vi "FPGA_HoppingStep_2ndEd(NoXYCalculation).vi"() -> ()   [LabVIEW 2014]
uses:
  <vilib>/Platform/TimedLoop/XDataNode/timing_clust.ctl
  <vilib>/Platform/TimedLoop/XDataNode/nitl_modes.ctl
  <vilib>/Platform/TimedLoop/XDataNode/wakeup.ctl
  <vilib>/rvi/Emulation/niFpgaGetClockAttributes.vi
  <vilib>/rvi/Emulation/niFpgaSctlEmulationGetInTimedLoop.vi
  <vilib>/rvi/Emulation/niFpgaEmulationReportErrorSimple.vi
  <vilib>/rvi/interface/RandomDataEmulation/niFpgaRandomDataHandleErrors.vi
  <vilib>/rvi/eio/common/nirviEmuTemplateMethod_errors.vi
  <vilib>/rvi/Emulation/niFpgaCriticalErrorInLSC.vi
  <vilib>/rvi/Emulation/niFpgaProcessEmulError.vi
  <vilib>/rvi/DataTransferAndStorage/Container/XNode/niFpgaContainer.xnode
  <vilib>/rvi/interface/RandomDataEmulation/nirviRandomDataFpgaReadWriteTemplate.vi
  <vilib>/eio/EIONode/EIONode.xnode
  <vilib>/Platform/TimedLoop/XDataNode/XDataNode.xnode
  <vilib>/Platform/TimedLoop/XDataNode/XDNodeRunTimeDep.lvlib
panel:
  out "LastObtained":i32(graph)
  in  "stop":bool
  out "Z":i32(graph)
  out "ZPresPos":i16
  in  "Sleep us":i16
  in  "RelativeWithdraw":i16
  in  "ZOffset":i16
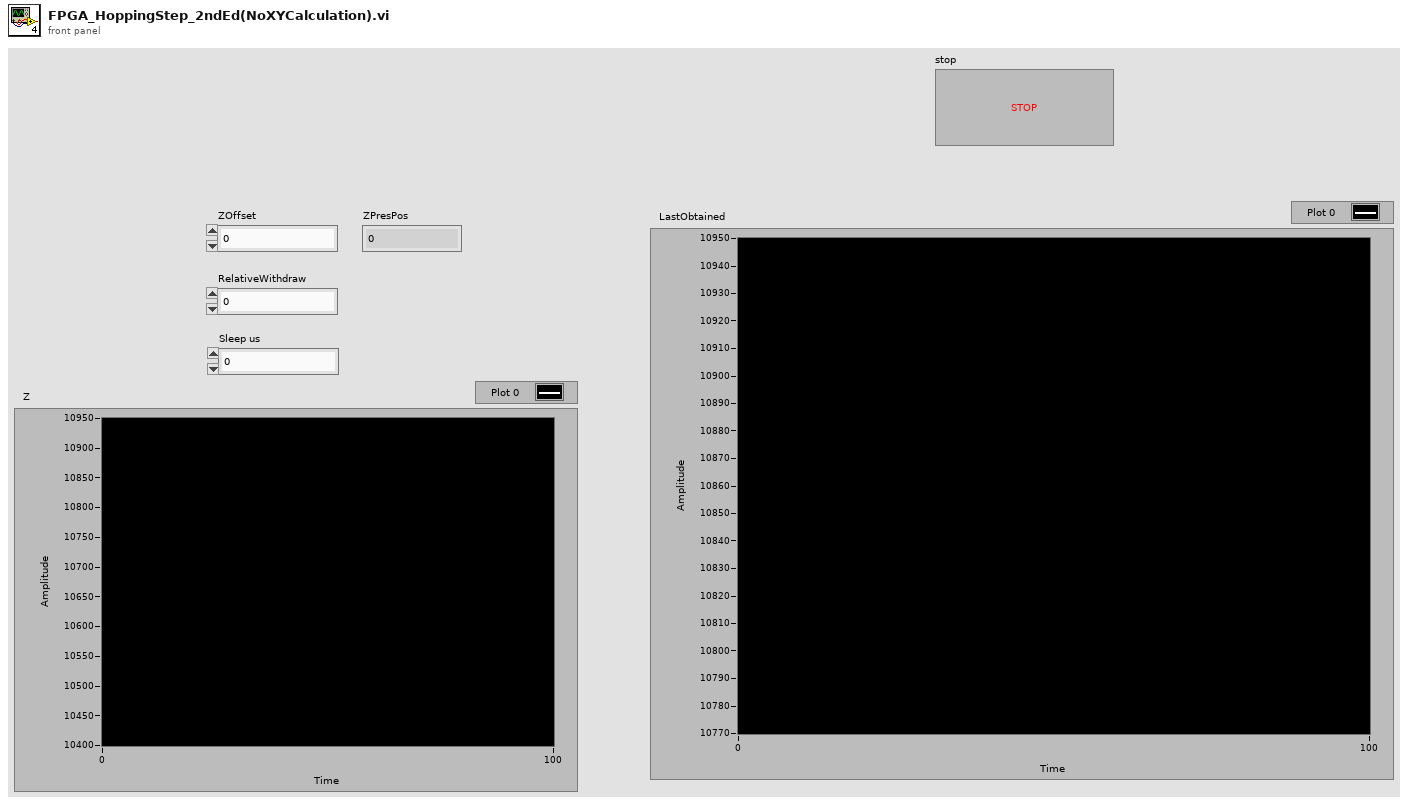
[diagram p1: front panel]
types:
  T1 = typedef "XDNodeRunTimeDep.lvlib/timing_clust.ctl" = cluster{"Expected End [f-1]":u64, "Actual End [f-1]":u64, "Finished Late? [f-1]":bool, "Expected End [i-1]":u64, "Actual End [i-1]":u64, "Finished Late? [i-1]":bool, "Expected Start [i]":u64, "Actual Start [i]":u64, "Expected Start [f]":u64, "Actual Start [f]":u64, "Source Name":string, "Structure Name":string, "Period":i64, "Deadline":i64, "Offset":i64, "Start":i64, "Priority":i32, "Timeout":i32, "Mode":T2, "Wakeup Reason":T3, "Error":errorcluster, "Source Type":string, "Secondary Source Type":string, "Global End Time":u64, "Global Start Time":u64, "Frame Duration":u64, "Iteration Duration":u64, "Assigned CPU":i32, "I/O Scan Engine Mode":u32}
  T2 = typedef "XDNodeRunTimeDep.lvlib/nitl_modes.ctl" = enum32{"No Change", "Process missed periods, maintain original phase", "Discard missed periods, maintain original phase", "Process missed periods, ignore original phase", "Discard missed periods, ignore original phase"}
  T3 = typedef "XDNodeRunTimeDep.lvlib/wakeup.ctl" = enum32{"Normal", "Aborted", "Asynchronous wakeup", "Timing source error", "Timed loop error", "Timeout"}
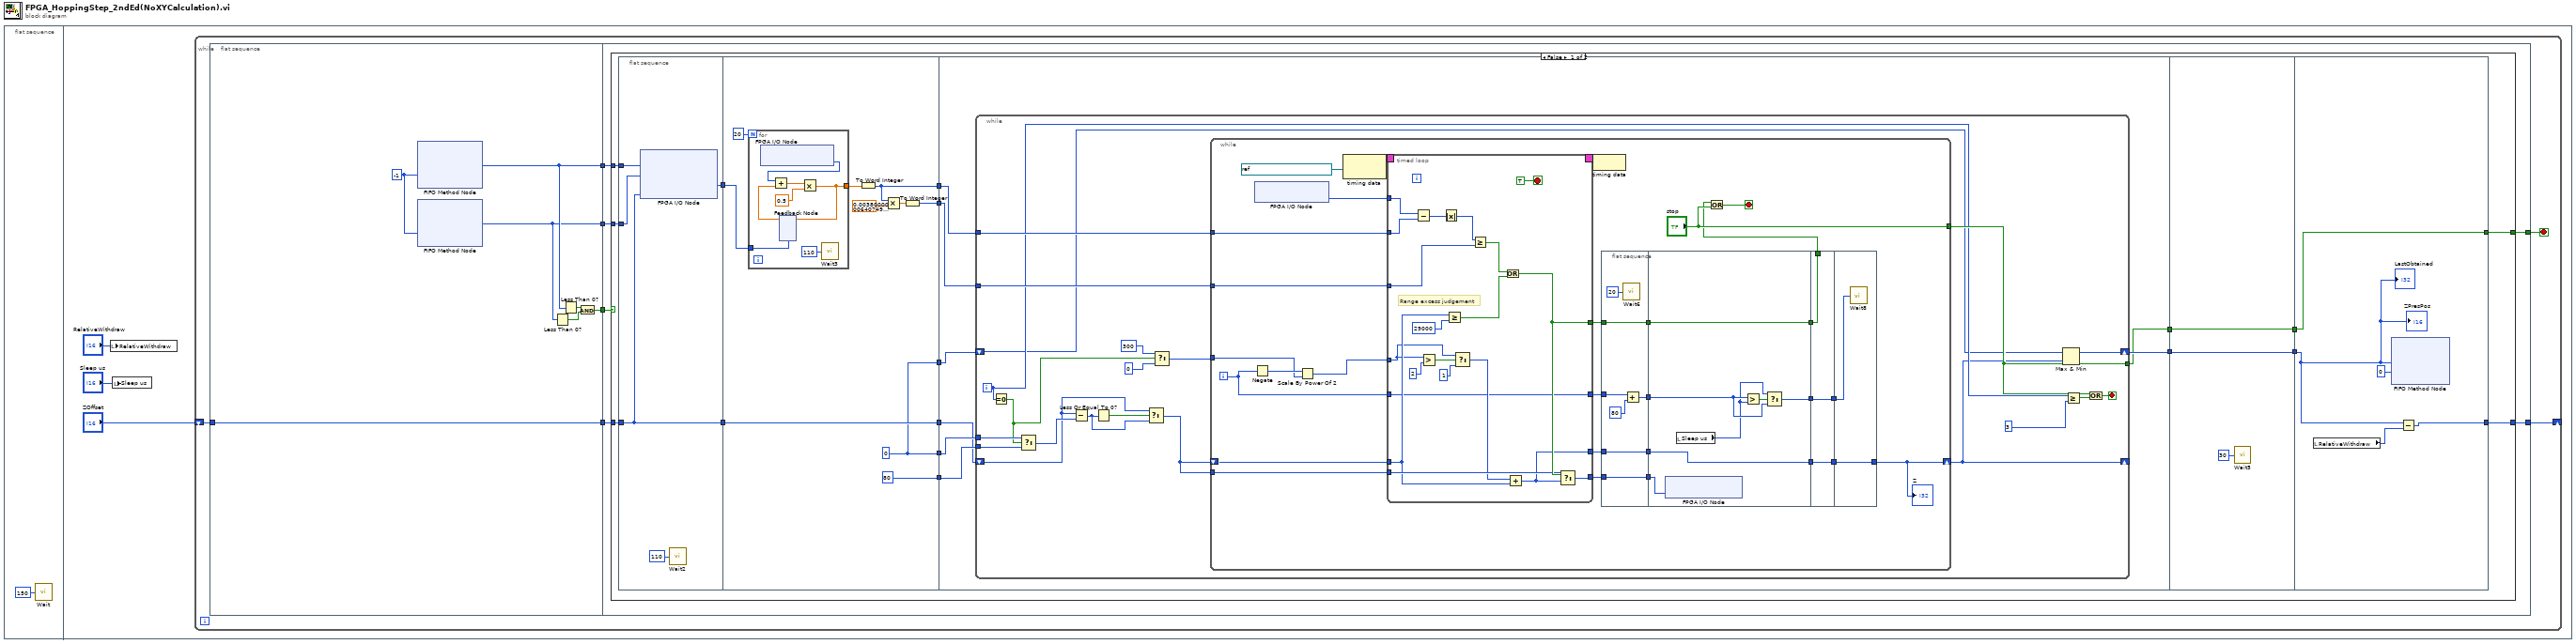
[diagram p0: block diagram]
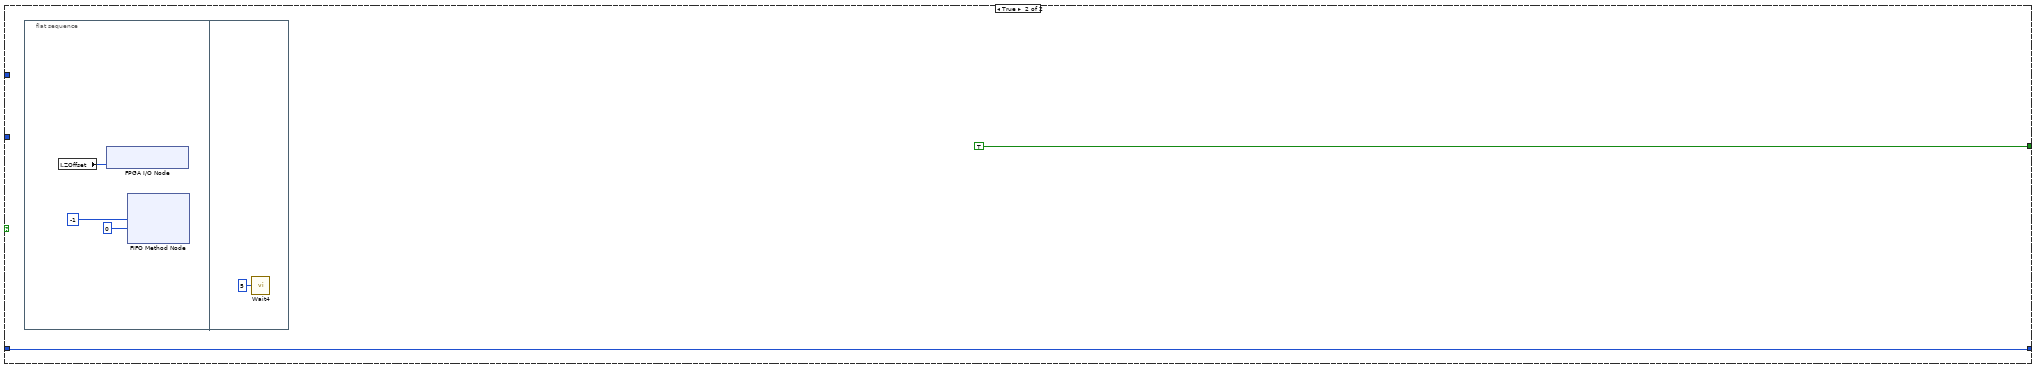
[diagram p2: hidden frame]
diagram:
  n1 = flat-sequence {
    frame #0 {
      n2 = call "Wait"("Count(mSec)"=u32 150) -> ()  [unwired: 1 out]
    }
    frame #1 {
      n3 = local write "RelativeWithdraw"("RelativeWithdraw") -> ()
      n4 = local write "Sleep us"("Sleep us") -> ()
      n5 = while {
        shift-right: [w6] -> _
        shift-left: "ZOffset" -> [w8]
        stop <- w5 stop-if-true
        n6 = flat-sequence {
          tunnel: [w18] -> w11
          tunnel: [w17] -> w10
          tunnel: [w14] -> w9
          tunnel: w8 -> [w13]
          tunnel: [w13] -> w7
          tunnel: w11 -> [w24]
          tunnel: w10 -> [w23]
          tunnel: w9 -> [w22]
          tunnel: w7 -> [w21]
          tunnel: [w20] -> w6
          tunnel: [w19] -> w5
          frame #0 {
            w12 = -1 ("Timeout")
            n7 = xnode ("FIFO Method Node")("Timeout"=w12) -> ("Element"=w18:i16)  [unwired: 1 in, 2 out]
            n8 = xnode ("FIFO Method Node")("Timeout"=w12) -> ("Element"=w17:i16)  [unwired: 1 in, 2 out]
            n9 = Less Than 0?(x=w17) -> (x < 0?=w15:bool)
            n10 = Less Than 0?(x=w18) -> (x < 0?=w16:bool)
            n11 = And(x=w16, y=w15) -> (x .and. y?=w14:bool)
          }
          frame #1 {
            n12 = case shown="False" w22 {
              tunnel: w24 -> [w41 _]
              tunnel: w23 -> [w40 _]
              tunnel: w21 -> [w39 w175]
              tunnel: [w31 TRUE ("stop")] -> w19
              tunnel: [w30 w175] -> w20
              frame False {
                n13 = flat-sequence {
                  tunnel: w41 -> [w46]
                  tunnel: w40 -> [w45]
                  tunnel: w39 -> [w42]
                  tunnel: [w42] -> w38
                  tunnel: [w43] -> w36
                  tunnel: w38 -> [w56]
                  tunnel: [w56] -> w37
                  tunnel: w36 -> [w48]
                  tunnel: [i16 80] -> w35
                  tunnel: [w49] -> w34
                  tunnel: [w52] -> w33
                  tunnel: [w50] -> w32
                  tunnel: [w50] -> w29
                  tunnel: w37 -> [w66]
                  tunnel: w35 -> [w68]
                  tunnel: w34 -> [w70]
                  tunnel: w33 -> [w71]
                  tunnel: w32 -> [w69]
                  tunnel: w29 -> [w67]
                  tunnel: [w65] -> w28
                  tunnel: [w64] -> w26
                  tunnel: w28 -> [w169]
                  tunnel: [w169] -> w27
                  tunnel: w26 -> [w168]
                  tunnel: [w168] -> w25
                  tunnel: [w171] -> w31
                  tunnel: [w172] -> w30
                  tunnel: w27 -> [w170]
                  tunnel: w25 -> [w171]
                  frame #0 {
                    n14 = xnode "FPGA I/O Node"("Connector0/AO2"=w46, "Connector0/AO3"=w45, "Connector0/AO0"=w42) -> ("Connector0/AI1"=w43:i16)  [unwired: 4 in, 4 out]
                    n15 = call "Wait2"("Count(uSec)"=u32 110) -> ()  [unwired: 1 out]
                  }
                  frame #1 {
                    w50 = i16 0
                    n16 = for {
                      N: 20 -> [_]
                      tunnel: w48 -> [w59]
                      tunnel: [w57] -> w47
                      n17 = xnode "FPGA I/O Node"() -> ("Connector0/AI1"=w62:i16)  [unwired: 1 in, 1 out]
                      n18 = feedback #1(w59) -> (w58:sgl)
                      n19 = Add(x=w62, y=w58) -> (x+y=w61:sgl)
                      n20 = Multiply(x=w61, y=sgl 0.5) -> (x*y=w57:sgl)
                      n21 = feedback-in #1(w57) -> ()
                      n22 = call "Wait3"("Count(uSec)"=u32 110) -> ()  [unwired: 1 out]
                    }
                    n23 = To Word Integer(number=w47) -> (16bit integer=w49:i16)
                    n24 = Multiply(x=w49, y=sgl 0.0038) -> (x*y=w53:sgl)
                    n25 = To Word Integer(number=w53) -> (16bit integer=w52:i16)
                  }
                  frame #2 {
                    n26 = while {
                      tunnel: w70 -> [w92]
                      tunnel: w71 -> [w91]
                      tunnel: [w88] -> w64
                      tunnel: w68 -> [w86]
                      shift-right: [w78] -> _
                      shift-left: w66 -> [w83]
                      tunnel: w67 -> [w80]
                      shift-right: [w77] -> w65
                      shift-left: w69 -> [w79]
                      i -> [w87]
                      stop <- w90 stop-if-true
                      n27 = Equal To 0?(x=w87) -> (x = 0?=w76:bool)
                      n28 = Select(t=w80, s=w76, f=w86) -> (s? t:f=w85:i16)
                      n29 = Subtract(x=w83, y=w85) -> (x-y=w82:i32)
                      n30 = Less Or Equal To 0?(x=w82) -> (x <= 0?=w84:bool)
                      n31 = Select(t=w83, s=w84, f=w82) -> (s? t:f=w81:i32)
                      n32 = Select(t=i16 300, s=w76, f=i16 0) -> (s? t:f=w73:i16)
                      n33 = while {
                        tunnel: w92 -> [w114]
                        tunnel: w91 -> [w116]
                        tunnel: ["stop"] -> w88
                        shift-right: [w106] -> w78
                        shift-left: w81 -> [w111]
                        tunnel: w81 -> [w108]
                        tunnel: w73 -> [w96]
                        i -> [w94]
                        stop <- w118 stop-if-true
                        n34 = Negate(x=w94) -> (-x=w97:i32)
                        n35 = xnode "FPGA I/O Node"() -> ("Connector0/AI1"=w115:i16)  [unwired: 1 in, 1 out]
                        n36 = Scale By Power Of 2(n=w97, x=w96) -> (x*2^n=w95:i16)
                        n37 = node-c288(refnum<k21> "40 MHz Onboard Clock" ("Source Name")) -> (w121:T1)
                        n38 = timed-loop {
                          timing: w121 -> [_]
                          timing-out: [_] -> w120
                          tunnel: w114 -> [w158]
                          tunnel: w116 -> [w142]
                          tunnel: w115 -> [w159]
                          tunnel: [w154] -> w112
                          tunnel: [w153] -> w110
                          tunnel: w111 -> [w150]
                          tunnel: w108 -> [w152]
                          tunnel: w95 -> [w145]
                          tunnel: [w147] -> w98
                          tunnel: w94 -> [w147]
                          tunnel: [w141] -> w93
                          stop <- TRUE stop-if-true
                          # "Range excess judgement"
                          n39 = Subtract(x=w159, y=w158) -> (x-y=w143:i16)
                          n40 = Greater?(x=w145, y=i16 2) -> (0:w144:bool)
                          n41 = Absolute Value(x=w143) -> (abs(x)=w157:i16)
                          n42 = Greater Or Equal?(x=w150, y=i16 29000) -> (x >= y?=w155:bool)
                          n43 = Select(t=w145, s=w144, f=1) -> (s? t:f=w148:i32)
                          n44 = Greater Or Equal?(x=w157, y=w142) -> (x >= y?=w156:bool)
                          n45 = Or(x=w156, y=w155) -> (x .or. y?=w153:bool)
                          n46 = Add(x=w148, y=w150) -> (x+y=w141:i32)
                          n47 = Select(t=w152, s=w153, f=w141) -> (s? t:f=w154:i32)
                        }
                        n48 = node-c288(w120) -> ()
                        n49 = flat-sequence {
                          tunnel: [w123] -> w113
                          tunnel: w112 -> [w123]
                          tunnel: w110 -> [w127]
                          tunnel: [w127] -> w109
                          tunnel: [w122] -> w107
                          tunnel: [w125] -> w99
                          tunnel: w98 -> [w126]
                          tunnel: w93 -> [w122]
                          tunnel: w113 -> [w133]
                          tunnel: [w135] -> w105
                          tunnel: w109 -> [w134]
                          tunnel: w107 -> [w135]
                          tunnel: [w134] -> w103
                          tunnel: [w131] -> w100
                          tunnel: w99 -> [w130]
                          tunnel: w105 -> [w138]
                          tunnel: [w138] -> w104
                          tunnel: w103 -> [w137]
                          tunnel: [w137] -> w102
                          tunnel: [w136] -> w101
                          tunnel: w100 -> [w136]
                          tunnel: w104 -> [w140]
                          tunnel: [w140] -> w106
                          tunnel: w101 -> [w139]
                          frame #0 {
                            n50 = call "Wait6"("Count(uSec)"=u32 20) -> ()  [unwired: 1 out]
                            n51 = Add(x=w126, y=80) -> (x+y=w125:i32)
                          }
                          frame #1 {
                            n52 = xnode "FPGA I/O Node"("Connector0/AO0"=w133) -> ()  [unwired: 1 in, 1 out]
                            n53 = local read "Sleep us"() -> (w129:i16)
                            n54 = Greater?(x=w130, y=w129) -> (0:w132:bool)
                            n55 = Select(t=w129, s=w132, f=w130) -> (s? t:f=w131:i32)
                          }
                          frame #2 {
                          }
                          frame #3 {
                            n56 = call "Wait8"("Count(uSec)"=w139) -> ()  [unwired: 1 out]
                          }
                        }
                        n57 = Or(x=w102, y="stop") -> (x .or. y?=w118:bool)
                        "Z" <- w106
                      }
                      n58 = Max & Min(x=w79, y=w78) -> (max(x,y)=w77:i32)  [unwired: 1 out]
                      n59 = Greater Or Equal?(x=w87, y=3) -> (x >= y?=w89:bool)
                      n60 = Or(x=w88, y=w89) -> (x .or. y?=w90:bool)
                    }
                  }
                  frame #3 {
                    n61 = call "Wait5"("Count(uSec)"=u32 30) -> ()  [unwired: 1 out]
                  }
                  frame #4 {
                    n62 = local read "RelativeWithdraw"() -> (w173:i16)
                    n63 = xnode ("FIFO Method Node")("Element"=w170, "Timeout"=0) -> ()  [unwired: 1 in, 2 out]
                    n64 = Subtract(x=w170, y=w173) -> (x-y=w172:i32)
                    "ZPresPos" <- w170
                    "LastObtained" <- w170
                  }
                }
              }
              frame True {
                n65 = flat-sequence {
                  frame #0 {
                    n66 = local read "ZOffset"() -> (w179:i16)
                    n67 = xnode "FPGA I/O Node"("Connector0/AO0"=w179) -> ()  [unwired: 1 in, 1 out]
                    n68 = xnode ("FIFO Method Node")("Element"=i16 -1, "Timeout"=0) -> ()  [unwired: 1 in, 2 out]
                  }
                  frame #1 {
                    n69 = call "Wait4"("Count(mSec)"=u32 5) -> ()  [unwired: 1 out]
                  }
                }
              }
            }
          }
        }
      }
    }
  }
